vi "CDMA_Channel.vi"(8 "error in (no error)":errorcluster caption="错误输入（无错误）", 10 "tx_data":cdb[](array[numeric]) format="%#_13g", 11 "Path":path) -> (0 "error out":errorcluster caption="错误输出", 2 "rx_data":cdb[](array[numeric]), 3 "Path Out":path)   [LabVIEW 2015]
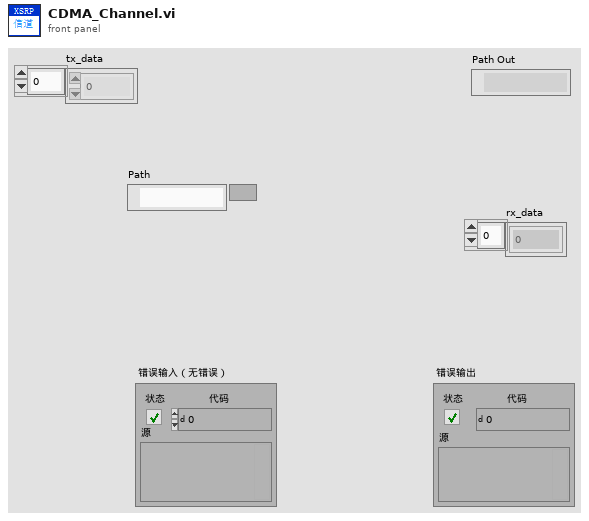
[diagram p1: front panel]
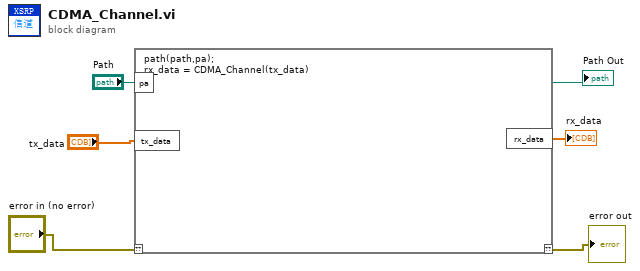
[diagram p0: block diagram]
diagram:
  n1 = script code="path(path,pa);\nrx_data = CDMA_Channel(tx_data)"("??"="error in (no error)", "pa"="Path", "tx_data"="tx_data") -> ("??"=→"error out":errorcluster, "rx_data"=→"rx_data":cdb[])
  "Path Out" <- "Path"
